vi "Self Test.vi"(8 "error in (no error)":errorcluster, 11 "Agilent 34401A in":refnum<class "Agilent 34401A.lvclass">) -> (0 "error out":errorcluster, 3 "Agilent 34401A out":refnum<class "Agilent 34401A.lvclass">)   [LabVIEW 2021, in "DMM.lvlib" / "Agilent 34401A.lvclass"]
uses:
  Agilent 34401A.lvclass
  Agilent 34401A.lvclass/Agilent 34401A.ctl
  <instrlib>/Agilent 34401/Agilent 34401.lvlib
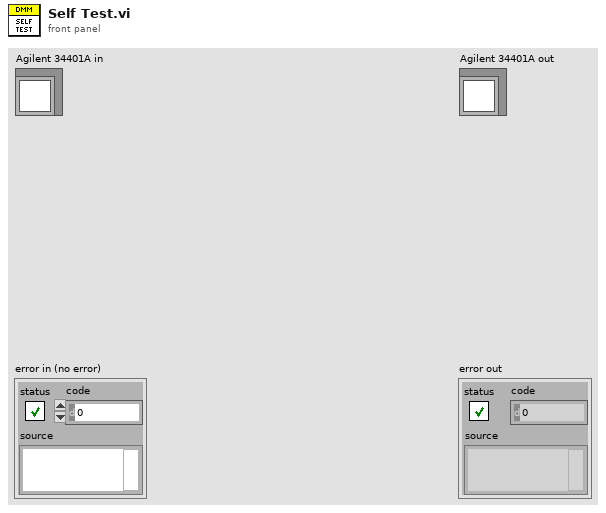
[diagram p1: front panel]
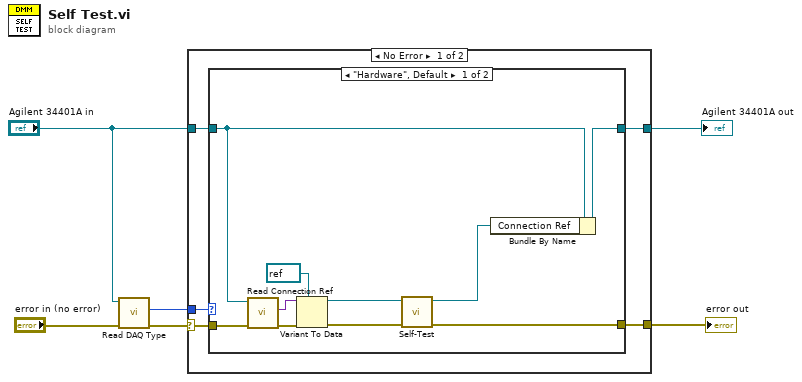
[diagram p0: block diagram]
diagram:
  n1 = call-dynamic "Read DAQ Type.vi"("error in (no error)"="error in (no error)", "Agilent 34401A in"="Agilent 34401A in") -> ("error out"=w5:errorcluster, "DAQ Type"=w4:enum16{"Hardware", "Simulation"})  [unwired: 7 in, 1 out]
  n2 = case shown="No Error" w5 {
    selector: w5 -> [w9 w24]
    tunnel: w4 -> [w11 _]
    tunnel: "Agilent 34401A in" -> [w10 w25]
    tunnel: [w8 w24] -> w2
    tunnel: [w7 w25] -> w1
    frame No Error {
      n3 = case shown="\"Hardware\", Default" w11 {
        tunnel: w10 -> [w14 w23]
        tunnel: w9 -> [w21 w22]
        tunnel: [w15 w22] -> w8
        tunnel: [w13 w23] -> w7
        frame "Hardware", Default {
          n4 = call-dynamic "Read Connection Ref.vi"("error in (no error)"=w21, "Agilent 34401A in"=w14) -> ("error out"=w20:errorcluster, "Connection Ref"=w19:variant)  [unwired: 7 in, 1 out]
          n5 = Variant To Data(error in=w20, type=refnum<visa-resource-name> refnum ("VISA resource name"), Variant=w19) -> (data=w17:refnum<visa-resource-name>, error out=w16:errorcluster)
          n6 = call <instrlib>:"Self-Test.vi"("error in (no error)"=w16, "VISA resource name"=w17) -> ("error out"=w15:errorcluster, "VISA resource name out"=w12:refnum<visa-resource-name>)  [unwired: 6 in, 2 out]
          n7 = Bundle By Name(cluster=w14, "Connection Ref"=w12) -> (w13:refnum<class "Agilent 34401A.lvclass">)
        }
        frame "Simulation" {
        }
      }
    }
    frame Error {
    }
  }
  "error out" <- w2
  "Agilent 34401A out" <- w1
